vi "SCMP - Read Cookbook.vi"(8 "error in":errorcluster, 10 "load preset cbk?":bool, 11 "preset cbk ring ref":refnum<vi>) -> (0 "error out":errorcluster, 1 "Recipe Files":string[](array[string]), 2 "# of Recipes":i16=9, 3 "Cookbook":T1=[{"Data Type"=enum."ACQUIRE DATA", "Arg 1"=0.0, "Arg 2"=0.0, "Arg 3"=path "", "Comments"=""}, {"Data Type"=enum."ACQUIRE DATA", "Arg 1"=0.0, "Arg 2"=0.0, "Arg 3"=path "", "Comments"=""}], 4 "min Cookbook Exposure [s]":dbl, 5 "Selected Cookbook":path, 6 "Cookbook Comments":string="\r")   [LabVIEW 2014]
uses:
  Controls/Cookbook.ctl
  Controls/Cbk Data type.ctl
  Controls/Globals.vi
  Controls/Global demo.vi
  <vilib>/Utility/file.llb/Read From Spreadsheet File (string).vi
  <vilib>/Utility/file.llb/Read From Spreadsheet File (DBL).vi
panel:
  out "Valid Check":bool[](array[boolean])=[TRUE, TRUE, TRUE, TRUE, TRUE, TRUE, TRUE, TRUE, TRUE]
  out "List of Recipes":path[](array[path])
  # "Arg 1 for a Filter Wheel is the desired position\nArg 1 for Set Exposure is the time in ms\nArg 1 for Acquire Data is the number of images to acquire"
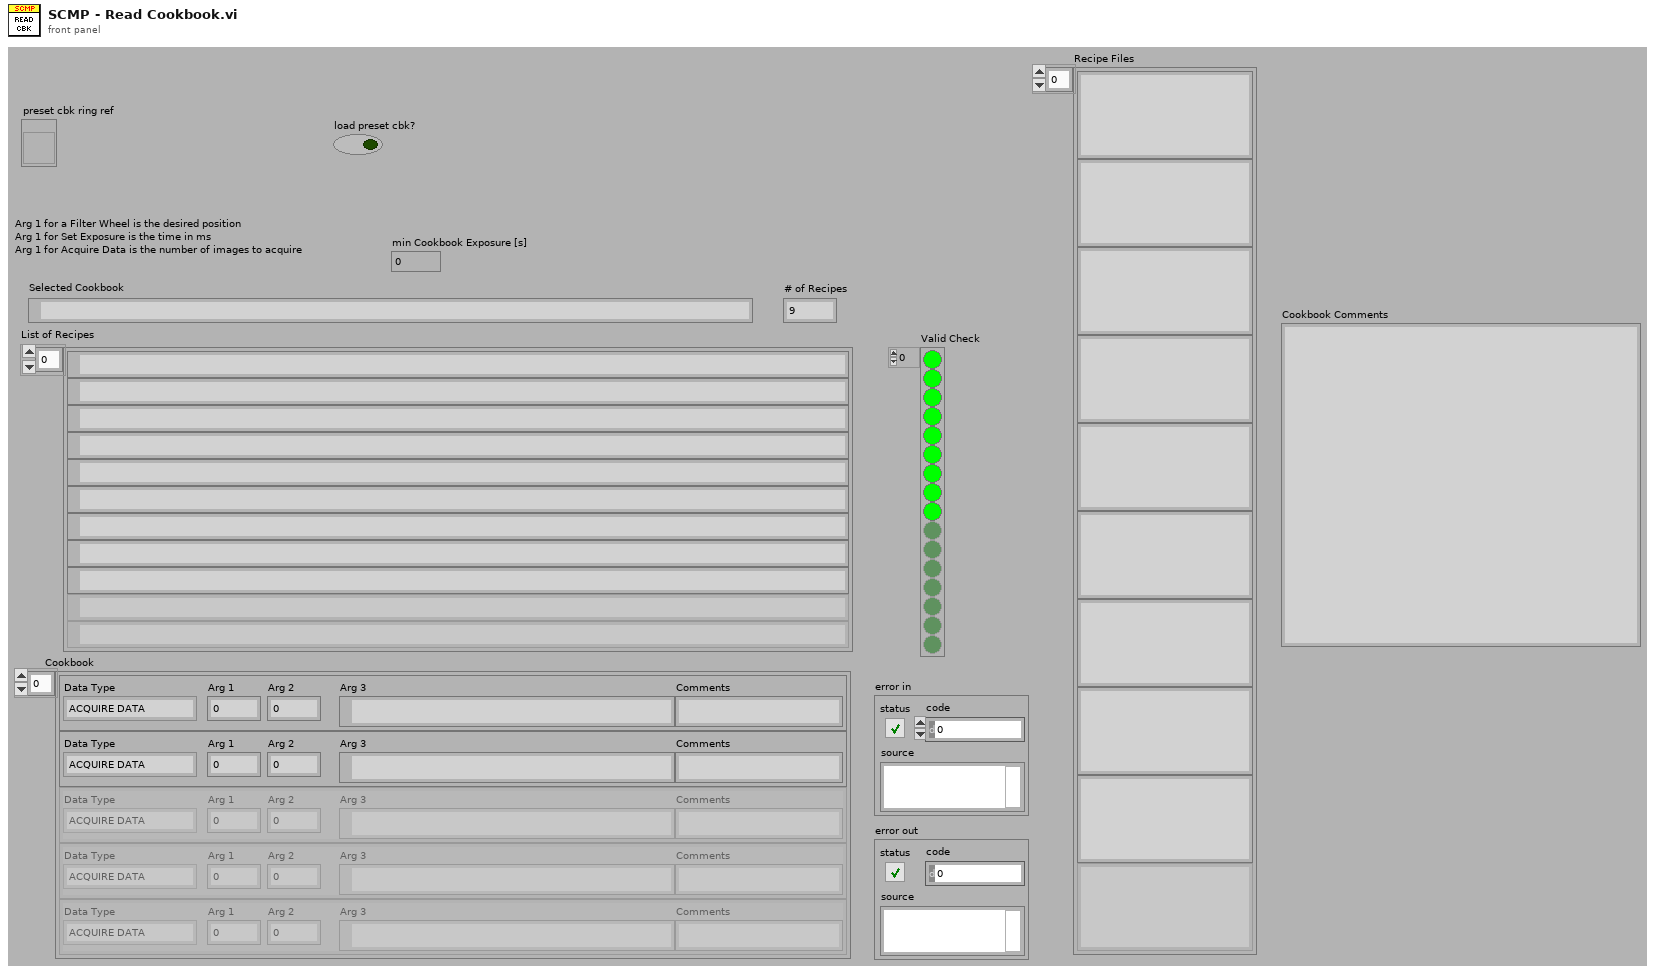
[diagram p1: front panel]
types:
  T1 = typedef "Cookbook.ctl" = cluster{"Data Type":T2, "Arg 1":sgl, "Arg 2":sgl, "Arg 3":path, "Comments":string}[]
  T2 = typedef "Cbk Data type.ctl" = enum32{"ACQUIRE DATA", "SET DIFFUSER", "CAL-FW", "WAVELENGTH-FW", "INSTR. ROTATION", "SET FOCUS", "DATATYPE", "SET EXPOSURE", "CBK COMMENTS", "MOVE-PI", "MOVE-PI2", "MOVE-PI3", "DWELL TIME", "BINNING"}
  T3 = cluster{"Data Type":T2, "Arg 1":sgl, "Arg 2":sgl, "Arg 3":path, "Comments":string}
  T4 = cluster{"Data Type":T2, "Arg 1":sgl, "Arg 2":sgl, "Arg 3":path, "Comments":string}[]
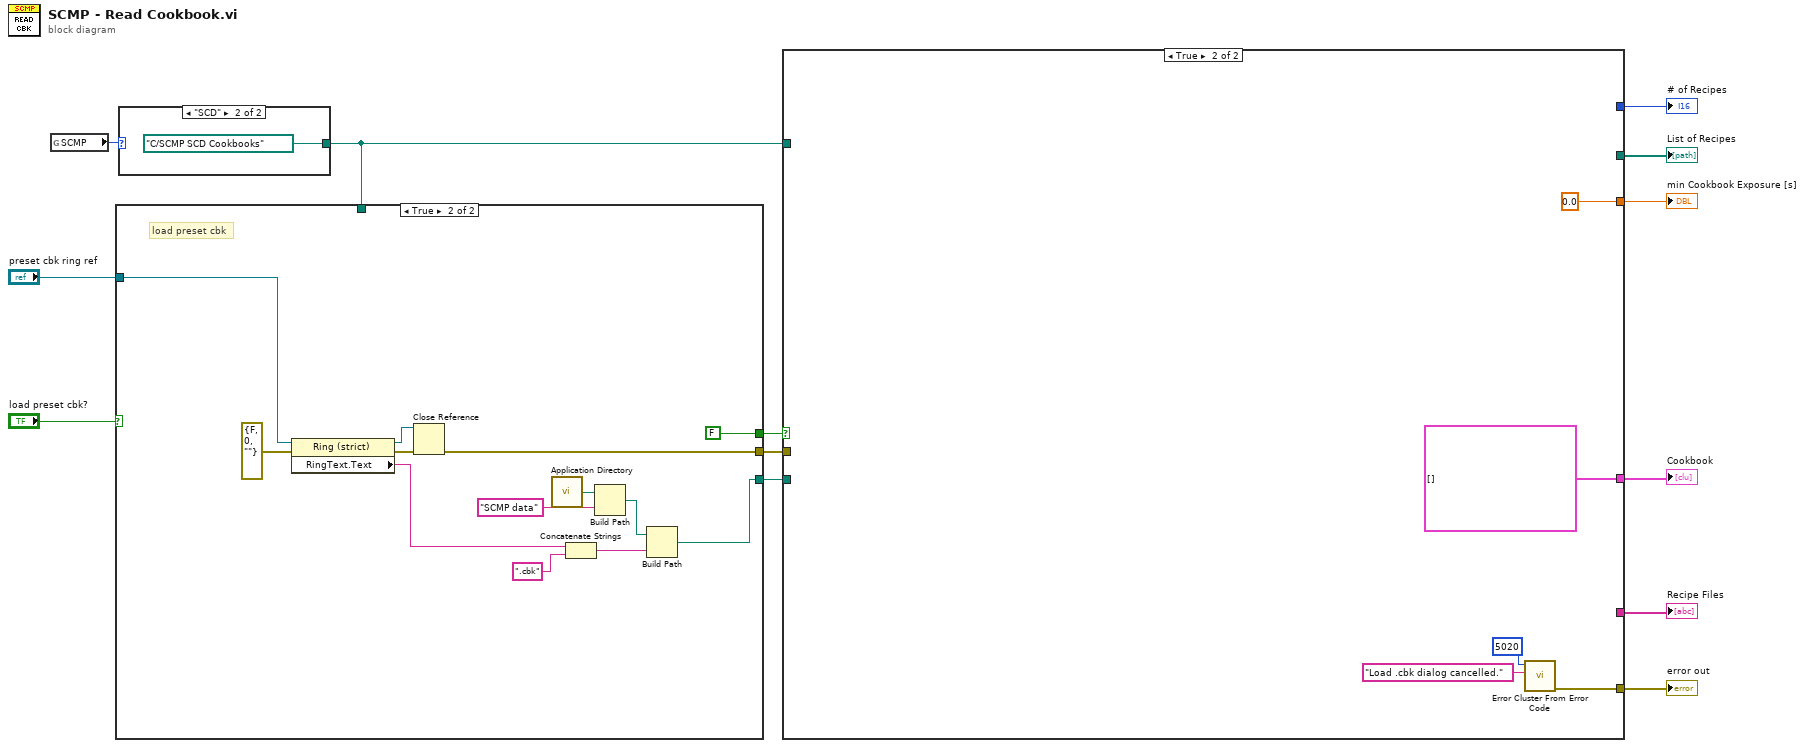
[diagram p0: block diagram]
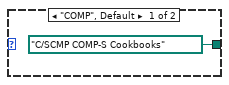
[diagram p2: hidden frame]
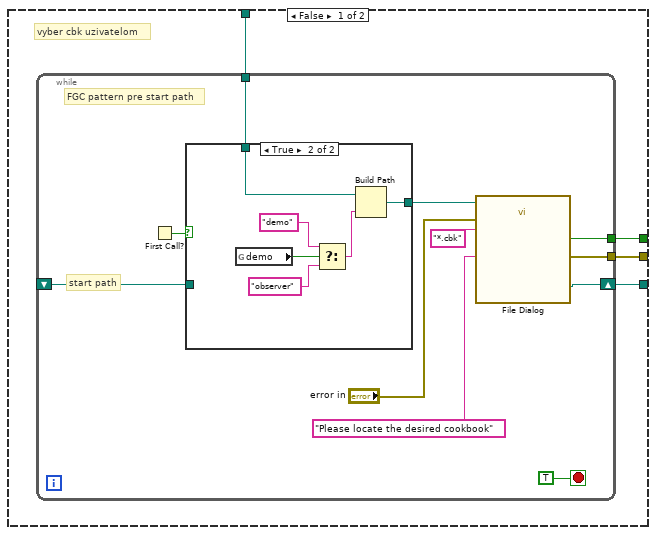
[diagram p3: hidden frame]
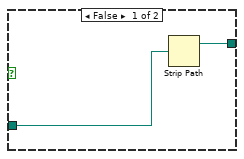
[diagram p4: hidden frame]
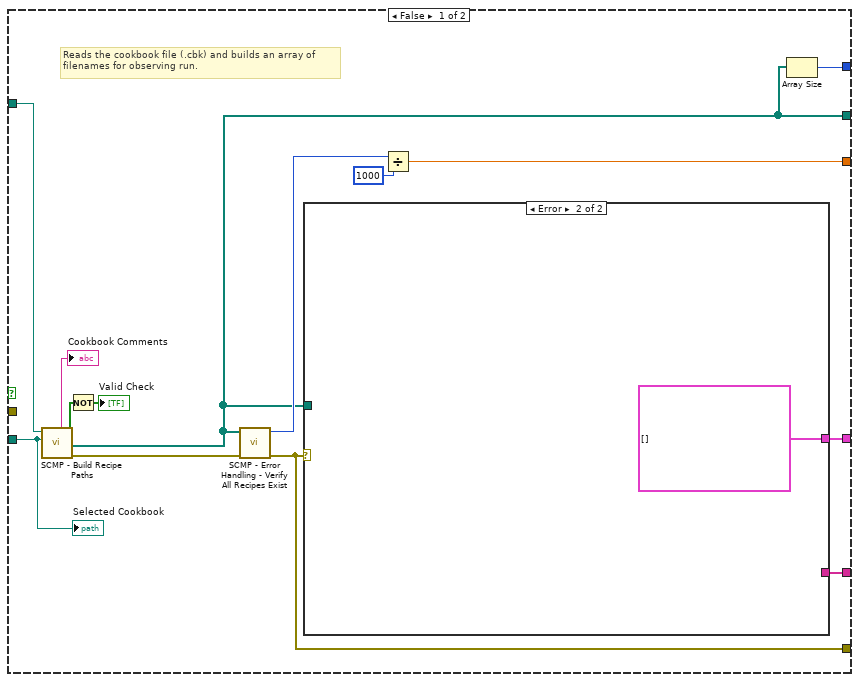
[diagram p5: hidden frame]
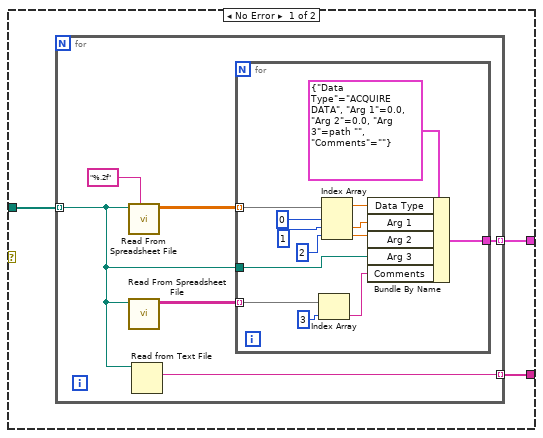
[diagram p6: hidden frame]
diagram:
  n1 = global read "Globals.vi" "SCMP"() -> (w3:enum16{"COMP", "SCD"})
  n2 = case shown="\"SCD\"" w3 {
    tunnel: [path "C:/SCMP COMP-S Cookbooks" ("COMP start path") path "C:/SCMP SCD Cookbooks" ("SCD start path")] -> w2
    frame "COMP", Default {
    }
    frame "SCD" {
    }
  }
  n3 = case shown="True" "load preset cbk?" {
    tunnel: [w19 w44] -> w13
    tunnel: [w18 FALSE ("cancelled")] -> w12
    tunnel: [w17 w45] -> w10
    tunnel: w2 -> [w16 _]
    tunnel: "preset cbk ring ref" -> [_ w42]
    frame False {
      # "vyber cbk uzivatelom"
      n4 = while {
        tunnel: [w28] -> w18
        tunnel: [w27] -> w17
        shift-right: [w22] -> w19
        shift-left: _ -> [w21]
        tunnel: w16 -> [w20]
        stop <- TRUE stop-if-true
        # "start path"
        # "FGC pattern pre start path"
        n5 = First Call?() -> (First Call?: T/F=w26:bool)
        n6 = case shown="True" w26 {
          tunnel: [w32 w38] -> w25
          tunnel: w21 -> [w31 _]
          tunnel: w20 -> [_ w33]
          frame False {
            n7 = Strip Path(path=w31) -> (stripped path=w32:path)  [unwired: 1 out]
          }
          frame True {
            n8 = global read "Global demo.vi" "demo"() -> (w36:bool)
            n9 = Select(t="demo" ("name or relative path"), s=w36, f="observer" ("name or relative path")) -> (s? t:f=w34:string)
            n10 = Build Path(base path=w33, name or relative path=w34) -> (appended path=w38:path)
          }
        }
        n11 = call "File Dialog"("start path"=w25, "prompt"="Please locate the desired cookbook", "error in"="error in", "pattern (all files)"="*.cbk") -> ("selected path"=w22:path, "cancelled"=w28:bool, "error out"=w27:errorcluster)  [unwired: 3 in, 6 out]
      }
    }
    frame True {
      # "load preset cbk"
      n12 = property class="Ring (strict)"(reference=w42, error in=errorcluster {"status"=FALSE, "code"=0, "source"=""} ("error out")) -> (reference out=w46:refnum<vi>, error out=w47:errorcluster, "RingText.Text"=w41:string)
      n13 = Close Reference(reference=w46, error in (no error)=w47) -> (error out=w45:errorcluster)
      n14 = call <vilib>:"Application Directory.vi"() -> ("Application Directory"=w50:path)
      n15 = Concatenate Strings(w41, ".cbk" ("string")) -> (w40:string)
      n16 = Build Path(base path=w50, name or relative path="SCMP data") -> (appended path=w49:path)
      n17 = Build Path(base path=w49, name or relative path=w40) -> (appended path=w44:path)
    }
  }
  n18 = case shown="True" w12 {
    tunnel: w13 -> [w63 _]
    tunnel: [w60 w91] -> w11
    tunnel: w10 -> [_ _]
    tunnel: w2 -> [w62 _]
    tunnel: [w57 T4 []] -> w9
    tunnel: [w55 _] -> w8
    tunnel: [w54 _] -> w6
    tunnel: [w53 0.0] -> w5
    tunnel: [w52 _] -> w4
    frame False {
      # "Reads the cookbook file (.cbk) and builds an array of\nfilenames for observing run."
      n19 = call "SCMP - Build Recipe Paths.vi"("Start path"=w62, "Selected Cookbook"=w63) -> ("Cookbook * Comments"=→"Cookbook Comments":string, "Recipe Not Found"=w59:bool[], "List of Recipes"=w54:path[], "error out"=w61:errorcluster)  [unwired: 5 in]
      n20 = Not(x=w59) -> (.not. x?=→"Valid Check":bool[])
      n21 = call "SCMP - Error Handling - Verify All Recipes Exist.vi"("error in (no error)"=w61, "List of Recipes"=w54) -> ("error out"=w60:errorcluster, "min Cookbook Exposure [ms]"=w56:i32)  [unwired: 6 in, 2 out]
      n22 = case shown="Error" w60 {
        tunnel: [w68 T4 []] -> w57
        tunnel: w54 -> [w67 _]
        tunnel: [w66 _] -> w55
        frame No Error {
          n23 = for {
            tunnel: w67 -> [w70] mode=indexing
            tunnel: [w72] -> w68 mode=indexing
            tunnel: [w69] -> w66 mode=indexing
            n24 = call-poly <vilib>:"Read From Spreadsheet File.vi"("format (%.3f)"="%.2f", "file path (dialog if empty)"=w70) -> ("all rows"=w74:dbl[][])  [unwired: 2 in, 7 out]
            n25 = call-poly <vilib>:"Read From Spreadsheet File.vi"("file path (dialog if empty)"=w70) -> ("all rows"=w71:string[][])  [unwired: 6 in, 4 out]
            n26 = Read from Text File(file (use dialog)=w70) -> (text=w69:string)  [unwired: 3 in, 3 out]
            n27 = for {
              tunnel: w74 -> [w87] mode=indexing
              tunnel: [w80] -> w72
              tunnel: w70 -> [w79]
              tunnel: w71 -> [w76] mode=indexing
              n28 = Index Array(array=w76, index=3) -> (element=w77:string)
              n29 = Index Array(array=w87, index #1=0 ("index"), index #2=1 ("index"), index #3=2 ("index")) -> (element #1=w83:dbl, element #2=w82:dbl, element #3=w81:dbl)
              n30 = Bundle By Name(cluster=T3 {"Data Type"=enum."ACQUIRE DATA", "Arg 1"=0.0, "Arg 2"=0.0, "Arg 3"=path "", "Comments"=""} ("element"), "Data Type"=w83, "Arg 1"=w82, "Arg 2"=w81, "Arg 3"=w79, "Comments"=w77) -> (w80:T3)
            }
          }
        }
        frame Error {
        }
      }
      n31 = Divide(x=w56, y=1000) -> (x/y=w53:dbl)
      n32 = Array Size(array=w54) -> (size(s)=w52:i32)
      "Selected Cookbook" <- w63
    }
    frame True {
      n33 = call <vilib>:"Error Cluster From Error Code.vi"("error message (\"\")"="Load .cbk dialog cancelled." ("message"), "error code (0)"=5020) -> ("error out"=w91:errorcluster)  [unwired: 7 in]
    }
  }
  "error out" <- w11
  "Cookbook" <- w9
  "Recipe Files" <- w8
  "List of Recipes" <- w6
  "min Cookbook Exposure [s]" <- w5
  "# of Recipes" <- w4
